vi "SubVI_Cam&Li_String.vi"(11 "Data String In":string) -> (3 "相機、光源":T1 {"光源亮度" step=1 scale=0.0..255.0; "相機選擇" items=["相機 1", "相機 2", "相機 3", "相機 4", "相機 5", "相機 6", "相機 7", "相機 8"]; "光源選擇" items=["光源 1", "光源 2", "光源 3", "光源 4", "光源 5", "光源 6", "光源 7", "光源 8"]})   [LabVIEW 2015]
uses:
  <userlib>/FGV/control/Control_Camera&Light.ctl
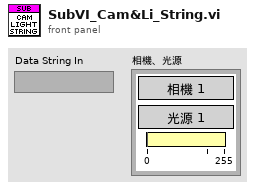
[diagram p1: front panel]
types:
  T1 = typedef "Control_Camera&Light.ctl" = cluster{"相機選擇":u8, "光源選擇":u16, "光源亮度":u8}
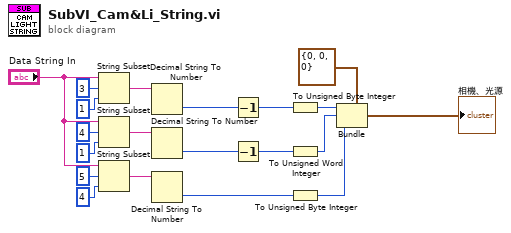
[diagram p0: block diagram]
diagram:
  n1 = String Subset(string="Data String In", offset (0)=3, length (rest)=1 ("length (rest)")) -> (substring=w13:string)
  n2 = String Subset(string="Data String In", offset (0)=4 ("length (rest)"), length (rest)=1 ("length (rest)")) -> (substring=w18:string)
  n3 = String Subset(string="Data String In", offset (0)=5 ("length (rest)"), length (rest)=4 ("length (rest)")) -> (substring=w19:string)
  n4 = Decimal String To Number(string=w13) -> (number=w3:i32)  [unwired: 2 in, 1 out]
  n5 = Decimal String To Number(string=w18) -> (number=w5:i32)  [unwired: 2 in, 1 out]
  n6 = Decimal String To Number(string=w19) -> (number=w1:i32)  [unwired: 2 in, 1 out]
  n7 = Decrement(x=w3) -> (x-1=w2:i32)
  n8 = Decrement(x=w5) -> (x-1=w4:i32)
  n9 = To Unsigned Byte Integer(number=w2) -> (unsigned 8bit integer=w10:u8)
  n10 = To Unsigned Word Integer(number=w4) -> (unsigned 16bit integer=w9:u16)
  n11 = To Unsigned Byte Integer(number=w1) -> (unsigned 8bit integer=w8:u8)
  n12 = Bundle(cluster=T1 {"相機選擇"=0, "光源選擇"=0, "光源亮度"=0} ("相機、光源"), "相機選擇"=w10, "光源選擇"=w9, "光源亮度"=w8) -> (→"相機、光源":T1)
